vi "clear menu.vi"(11 "Menu in":refnum<k9>) -> (0 "error out":errorcluster, 3 "Menu out":refnum<k9>)   [LabVIEW 2013, in "fixed channel tag bus module editor node.lvclass"]
uses:
  fixed channel tag bus module editor node.lvclass
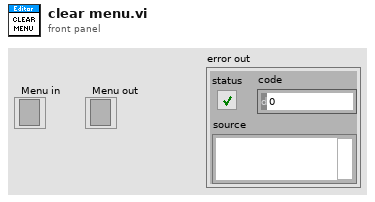
[diagram p1: front panel]
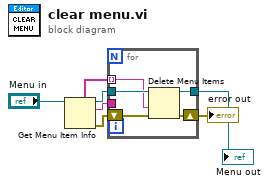
[diagram p0: block diagram]
diagram:
  n1 = Get Menu Item Info(11:"Menu in") -> (0:w2:errorcluster, 2:w4:string, 3:w5:refnum<k9>, 5:w6:string[])  [unwired: 2 in, 3 out]
  n2 = for {
    tunnel: w6 -> [w11] mode=indexing
    tunnel: w5 -> [w12]
    tunnel: w4 -> [_]
    tunnel: [w10] -> w3
    shift-right: [w8] -> w1
    shift-left: w2 -> [w9]
    n3 = Delete Menu Items(6:w9, 7:w11, 9:w12) -> (0:w8:errorcluster, 3:w10:refnum<k9>)  [unwired: 1 in]
  }
  "Menu out" <- w3
  "error out" <- w1
